vi "Color array_out of range_deleteafterjuly.vi"(9 "Number of sensors":i32, 10 "Array to specify\nthe range":dbl[][](array[numeric]), 11 "Input Array":string[](array[string])) -> (0 "Data from arduino in range?":bool[](array[boolean]), 3 "output array with color code":cluster{"Color Box":u32, "String":string}[](array[cluster]))   [LabVIEW 2012]
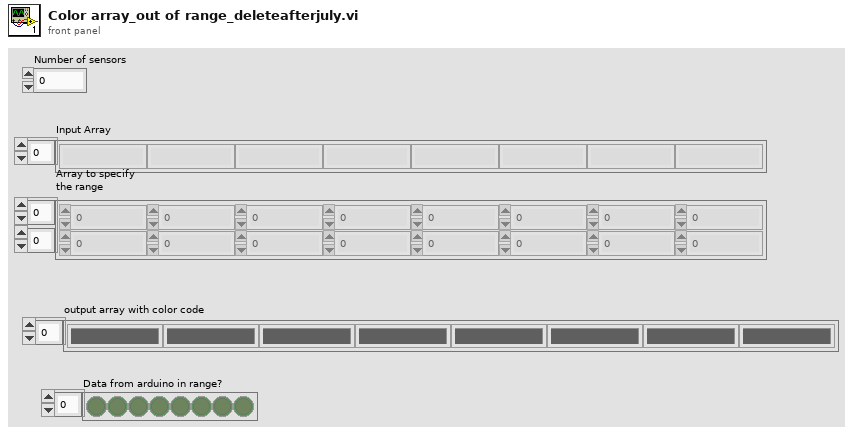
[diagram p1: front panel]
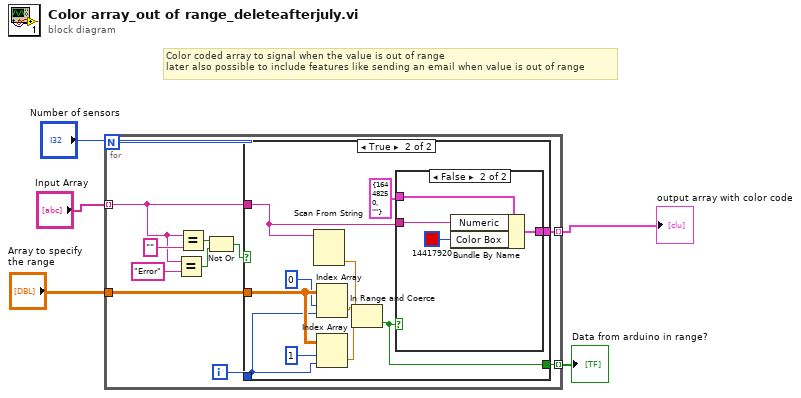
[diagram p0: block diagram]
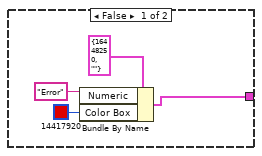
[diagram p2: hidden frame]
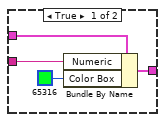
[diagram p3: hidden frame]
diagram:
  # "Color coded array to signal when the value is out of range\nlater also possible to include features like sending an email when value is out of range"
  n1 = for {
    N: "Number of sensors" -> [_]
    tunnel: [w15] -> w5 mode=indexing
    tunnel: "Array to specify\nthe range" -> [w14]
    tunnel: "Input Array" -> [w8] mode=indexing
    tunnel: [w6] -> w1 mode=indexing
    i -> [w13]
    n2 = Equal?(x=w8, y="Error") -> (x = y?=w9:bool)
    n3 = Equal?(x=w8, y="") -> (x = y?=w11:bool)
    n4 = Not Or(1:w9, 2:w11) -> (0:w10:bool)
    n5 = case shown="True" w10 {
      tunnel: [w17 w29] -> w15
      tunnel: w14 -> [_ w26]
      tunnel: w8 -> [_ w21]
      tunnel: w13 -> [_ w22]
      tunnel: [_ w20] -> w6
      frame False {
        n6 = Bundle By Name(cluster=cluster{"Color Box":u32, "Numeric":string} {"Color Box"=16448250, "Numeric"=""} ("Cluster"), "Numeric"="Error", "Color Box"=u32 14417920) -> (w17:cluster{"Color Box":u32, "Numeric":string})
      }
      frame True {
        n7 = Scan From String(input string=w21) -> (output 1=w23:dbl)  [unwired: 4 in, 3 out]
        n8 = Index Array(array=w26, index (row)=0, index (col)=w22) -> (element=w28:dbl)
        n9 = Index Array(array=w26, index (row)=1 ("disabled index (row)"), index (col)=w22) -> (element=w27:dbl)
        n10 = In Range and Coerce(upper limit=w28, x=w23, lower limit=w27) -> (In Range?=w20:bool)  [unwired: 1 out]
        n11 = case shown="False" w20 {
          tunnel: cluster{"Color Box":u32, "Numeric":string} {"Color Box"=16448250, "Numeric"=""} ("Cluster") -> [w34 w38]
          tunnel: [w33 w37] -> w29
          tunnel: w21 -> [w32 w35]
          frame True {
            n12 = Bundle By Name(cluster=w34, "Numeric"=w32, "Color Box"=u32 65316) -> (w33:cluster{"Color Box":u32, "Numeric":string})
          }
          frame False {
            n13 = Bundle By Name(cluster=w38, "Numeric"=w35, "Color Box"=u32 14417920) -> (w37:cluster{"Color Box":u32, "Numeric":string})
          }
        }
      }
    }
  }
  "output array with color code" <- w5
  "Data from arduino in range?" <- w1
